vi "joysticki.vi"(9 "Multicolumn Listbox":i32(listbox), 10 "stop":bool) -> (11 "Numeric":i32)   [LabVIEW 2015]
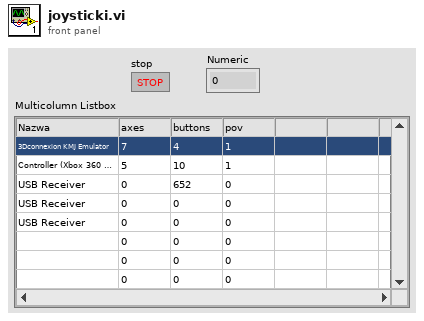
[diagram p1: front panel]
types:
  T1 = cluster{"axes total":u32, "buttons total":u32, "pov total":u32, "device name":string}[]
  T2 = cluster{"axes total":u32, "buttons total":u32, "pov total":u32, "device name":string}
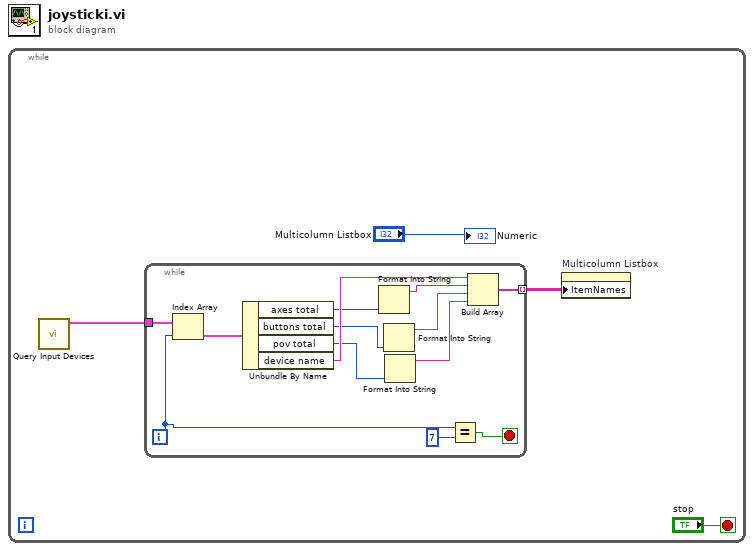
[diagram p0: block diagram]
diagram:
  n1 = while {
    stop <- "stop" stop-if-true
    n2 = call <vilib>:"Query Input Devices.vi"() -> ("joystick info"=w4:T1)  [unwired: 8 in, 3 out]
    n3 = while {
      tunnel: w4 -> [w17]
      tunnel: [w15] -> w2 mode=indexing
      i -> [w5]
      stop <- w7 stop-if-true
      n4 = Index Array(array=w17, index=w5) -> (element=w16:T2)
      n5 = Unbundle By Name(w16) -> ("axes total"=w8:u32, "buttons total"=w12:u32, "pov total"=w11:u32, "device name"=w14:string)
      n6 = Format Into String(w8) -> (resulting string=w13:string)  [unwired: 3 in, 1 out]
      n7 = Format Into String(w12) -> (resulting string=w10:string)  [unwired: 3 in, 1 out]
      n8 = Format Into String(w11) -> (resulting string=w9:string)  [unwired: 3 in, 1 out]
      n9 = Equal?(x=w5, y=7) -> (x = y?=w7:bool)
      n10 = Build Array(w14, w13, w10, w9) -> (w15:string[])
    }
    n11 = property on="Multicolumn Listbox" class="MCListbox (strict)"("ItemNames"=w2) -> ()  [unwired: 2 in, 2 out]
    "Numeric" <- "Multicolumn Listbox"
  }
